vi "Update Method Results.vi"(8 "error in (no error)":errorcluster, 10 "Method Result":T1, 11 "Result Table in":refnum<class "Result Table V2.lvclass">) -> (0 "error out":errorcluster, 3 "Result Table out":refnum<class "Result Table V2.lvclass">)   [LabVIEW 2020, in "Result Table V2.lvclass"]
uses:
  Result Table V2.lvclass
  Framework/Result Types/Assertion Result/Public/TypeDefs/Status.ctl
  Result Table V2.lvclass/Result Table V2.ctl
  Framework/Result Types/Assertion Result/Assertion Result.lvlib
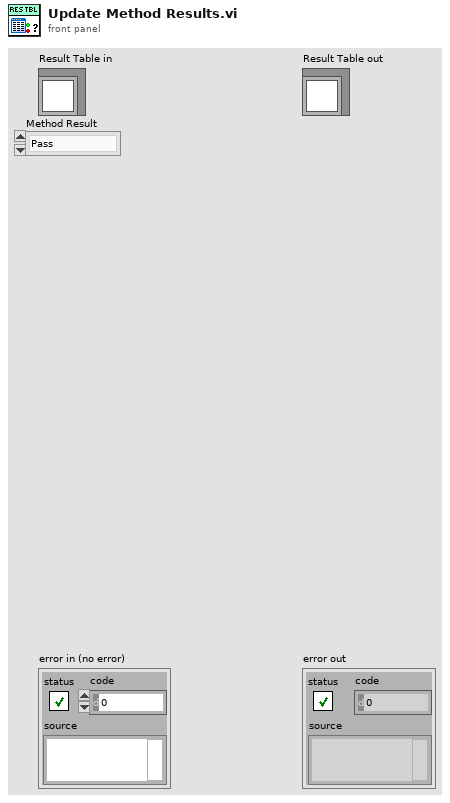
[diagram p1: front panel]
types:
  T1 = typedef "Assertion Result.lvlib/Status.ctl" = enum16{"Pass", "Fail", "Error", "Skipped", "Setup Error", "Broken", "Teardown Error"}
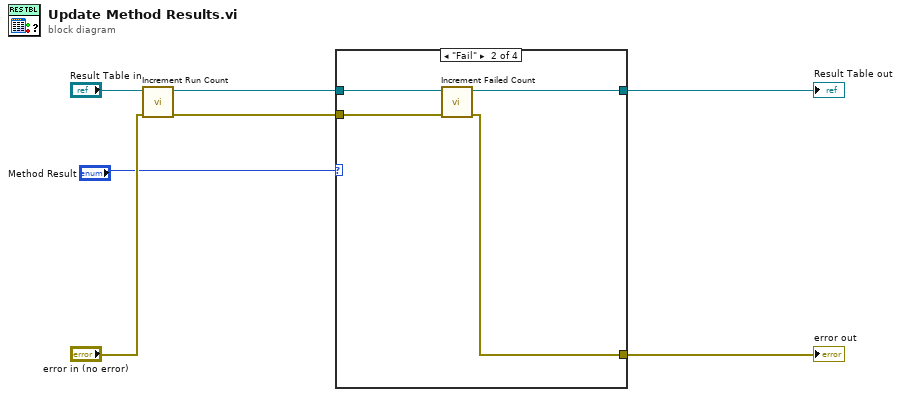
[diagram p0: block diagram]
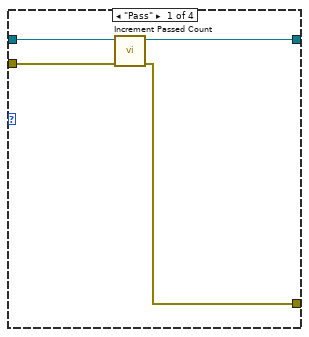
[diagram p2: hidden frame]
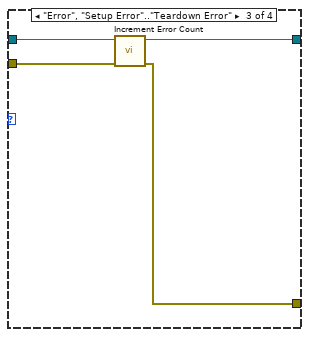
[diagram p3: hidden frame]
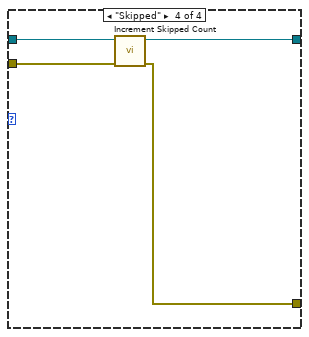
[diagram p4: hidden frame]
diagram:
  n1 = call "Increment Run Count.vi"("error in (no error)"="error in (no error)", "Result Table.lvclass"="Result Table in") -> ("error out"=w3:errorcluster, "Result Table"=w5:refnum<class "Result Table V2.lvclass">)  [unwired: 8 in]
  n2 = case shown="\"Fail\"" "Method Result" {
    tunnel: w5 -> [w11 w15 w19 w23]
    tunnel: [w10 w14 w18 w22] -> w2
    tunnel: [w9 w13 w17 w21] -> w7
    tunnel: w3 -> [w8 w12 w16 w20]
    frame "Pass" {
      n3 = call "Increment Passed Count.vi"("error in (no error)"=w8, "Result Table.lvclass"=w11) -> ("error out"=w9:errorcluster, "Result Table"=w10:refnum<class "Result Table V2.lvclass">)  [unwired: 8 in]
    }
    frame "Fail" {
      n4 = call "Increment Failed Count.vi"("error in (no error)"=w12, "Result Table.lvclass"=w15) -> ("error out"=w13:errorcluster, "Result Table"=w14:refnum<class "Result Table V2.lvclass">)  [unwired: 8 in]
    }
    frame "Error", "Setup Error".."Teardown Error" {
      n5 = call "Increment Error Count.vi"("error in (no error)"=w16, "Result Table.lvclass"=w19) -> ("error out"=w17:errorcluster, "Result Table"=w18:refnum<class "Result Table V2.lvclass">)  [unwired: 8 in]
    }
    frame "Skipped" {
      n6 = call "Increment Skipped Count.vi"("error in (no error)"=w20, "Result Table.lvclass"=w23) -> ("error out"=w21:errorcluster, "Result Table"=w22:refnum<class "Result Table V2.lvclass">)  [unwired: 8 in]
    }
  }
  "error out" <- w7
  "Result Table out" <- w2
